vi "Initialize.vi"(7 "menu ref":refnum<k9>, 8 "error in":errorcluster, 11 "class objects IN":T1) -> (0 "error out":errorcluster, 3 "class objects OUT":T1)   [LabVIEW 2011]
uses:
  Controls/Class Objects.ctl
  Modules/File/Configuration/Configuration.lvclass
  Modules/Hardware/Power Supply/Power Supply.lvclass
  Modules/Hardware/Mass Flow Controller/Mass Flow Controller.lvclass
  Modules/Hardware/Detector/Detector.lvclass
  Modules/File/TDMS/TDMS.lvclass
  Functional Globals/Device Parameters.ctl
  Modules/File/Configuration/File Type.ctl
  Controls/Class Labels.ctl
  Modules/Menu/Menu Action.ctl
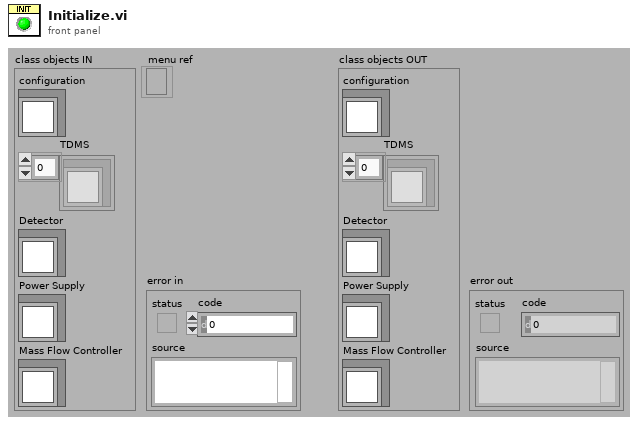
[diagram p1: front panel]
types:
  T1 = typedef "Class Objects.ctl" = cluster{"configuration":refnum<class "Configuration.lvclass">, "TDMS":refnum<class "TDMS.lvclass">[], "Power Supply":refnum<class "Power Supply.lvclass">, "Mass Flow Controller":refnum<class "Mass Flow Controller.lvclass">, "Detector":refnum<class "Detector.lvclass">}
  T2 = typedef "Device Parameters.ctl" = enum16{"Initialize", "Set Device Connections", "Set Device Settings", "Get Device Connections", "Get Device Settings"}
  T3 = typedef "Configuration.lvclass/File Type.ctl" = enum16{"INI", "XML"}
  T4 = typedef "Class Labels.ctl" = enum16{"Configuration", "TDMS", "Detector", "Power Supply", "MFC", "NMR", "Valve Controller"}
  T5 = typedef "Menu Action.ctl" = enum16{"Initialize", "Insert Item", "Remove Item", "Set Checked Item", "Get Checked Item", "Get Item Index", "Item Present?", "Stop"}
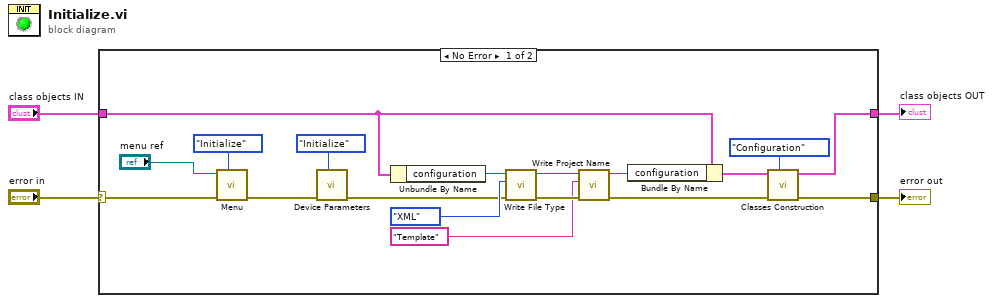
[diagram p0: block diagram]
diagram:
  n1 = case shown="No Error" "error in" {
    selector: "error in" -> [w20 w24]
    tunnel: [w18 w24] -> w3
    tunnel: "class objects IN" -> [w12 w23]
    tunnel: [w8 w23] -> w1
    frame No Error {
      n2 = call "Menu.vi"("action"=Menu_Action."Initialize" ("Menu"), "error in"=w20, "menu reference"="menu ref") -> ("error out"=w7:errorcluster)  [unwired: 5 in, 3 out]
      n3 = call "Device Parameters.vi"("command"=Device_Parameters."Initialize", "error in"=w7) -> ("error out"=w6:errorcluster)  [unwired: 7 in, 2 out]
      n4 = Unbundle By Name(w12) -> ("configuration"=w17:refnum<class "Configuration.lvclass">)
      n5 = call-dynamic "Write File Type.vi"("error in (no error)"=w6, "File Type"=File_Type."XML", "Configuration in"=w17) -> ("error out"=w15:errorcluster, "Configuration out"=w14:refnum<class "Configuration.lvclass">)  [unwired: 7 in]
      n6 = call-dynamic "Write Project Name.vi"("error in (no error)"=w15, "Project Name"="Template", "Configuration in"=w14) -> ("error out"=w10:errorcluster, "Configuration out"=w11:refnum<class "Configuration.lvclass">)  [unwired: 7 in]
      n7 = Bundle By Name(cluster=w12, "configuration"=w11) -> (w9:T1)
      n8 = call "Classes Construction.vi"("class"=Class_Labels."Configuration" ("Enum"), "error in"=w10, "classes in"=w9) -> ("error out"=w18:errorcluster, "classes out"=w8:T1)  [unwired: 5 in, 1 out]
    }
    frame Error {
    }
  }
  "error out" <- w3
  "class objects OUT" <- w1
